vi "optimize swerve.vi"(8 "error in (no error)":errorcluster, 9 "current angle (deg)":dbl, 10 "target angle (deg)":dbl, 11 "velocity":dbl) -> (0 "error out":errorcluster, 1 "reset POS to ABS":bool, 2 "steer angle (deg)":dbl=-90.0, 3 "velocity":dbl)   [LabVIEW 2023]
uses:
  <vilib>/Analysis/coordinate.llb/Angle Units.ctl
  <vilib>/Analysis/coordinate.llb/Angle Range (Degree).ctl
  <vilib>/Analysis/coordinate.llb/Wrap Angle (scalar).vi
  <vilib>/Analysis/NI_AAL_Angle.lvlib
panel:
  out "invert V":bool
  out "angle to supp":dbl=-90.0
  out "angle to target":dbl=90.0
  out "supp angle":dbl=-90.0
  out "angle delta CCW":dbl=90.0
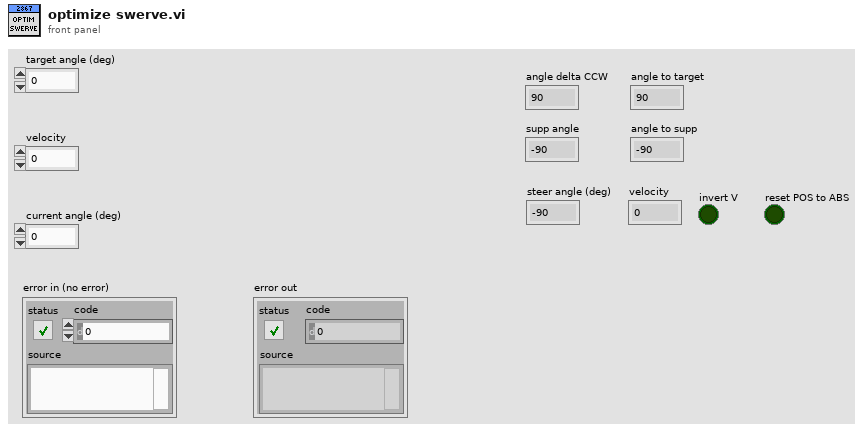
[diagram p1: front panel]
types:
  T1 = typedef "NI_AAL_Angle.lvlib/Angle Range (Degree).ctl" = u16
  T2 = typedef "NI_AAL_Angle.lvlib/Angle Units.ctl" = i32
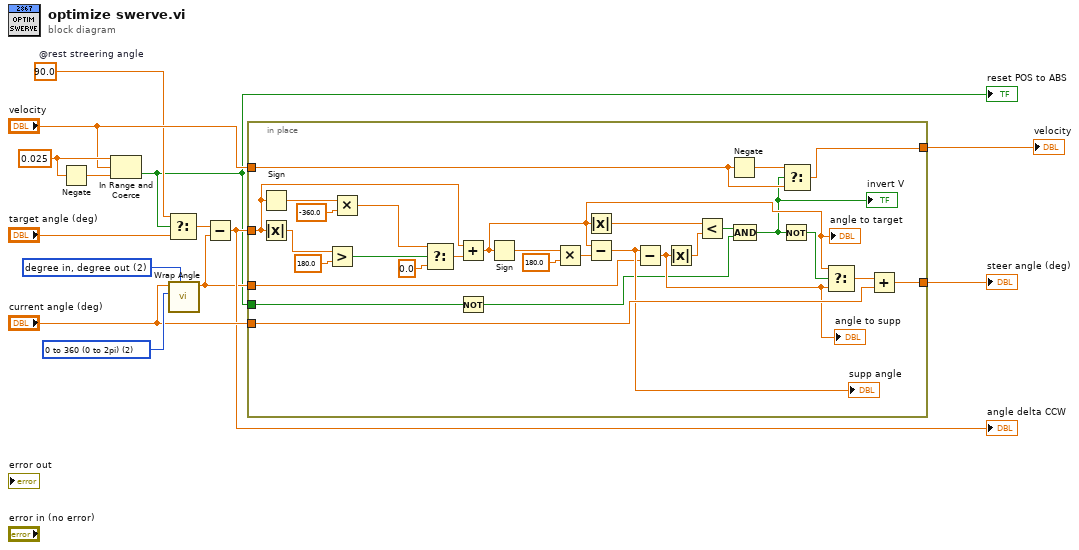
[diagram p0: block diagram]
diagram:
  w2 = 90.0  # @rest streering angle
  w5 = 0.025 ("upper limit")
  w12 = T1 2 items=["none", "-180 to 180 (-pi to pi)", "0 to 360 (0 to 2pi)"] ("angle range")
  w13 = T2 2 items=["radian in, radian out", "radian in, degree out", "degree in, degree out", "degree in, radian out"] ("angle units")
  n1 = Negate(x=w5) -> (-x=w4:dbl)
  n2 = In Range and Coerce(upper limit=w5, x="velocity", lower limit=w4) -> (In Range?=w1:bool)  [unwired: 1 out]
  "reset POS to ABS" <- w1
  n3 = Select(t=w2, s=w1, f="target angle (deg)") -> (s? t:f=w6:dbl)
  n4 = call-poly <vilib>:"Wrap Angle.vi"("angle units"=w13, "angle range"=w12, "angle in"="current angle (deg)") -> ("angle out"=w8:dbl)  [unwired: 7 in, 1 out]
  n5 = Subtract(x=w6, y=w8) -> (x-y=w10:dbl)
  "angle delta CCW" <- w10
  n6 = in-place {
    in-place-border: w10 -> [w38]
    in-place-border: "current angle (deg)" -> [w34]
    in-place-border: [w25] -> w14
    in-place-border: w8 -> [w31]
    in-place-border: [w21] -> w7
    in-place-border: "velocity" -> [w20]
    in-place-border: w1 -> [w18]
    n7 = Sign(1:w38) -> (0:w37:dbl)
    n8 = Absolute Value(x=w38) -> (abs(x)=w43:dbl)
    n9 = Greater?(x=w43, y=180.0) -> (0:w41:bool)
    n10 = Multiply(x=w37, y=-360.0 ("t")) -> (x*y=w36:dbl)
    n11 = Select(t=w36, s=w41, f=0.0) -> (s? t:f=w39:dbl)
    n12 = Add(x=w38, y=w39) -> (x+y=w24:dbl)
    "angle to target" <- w24
    n13 = Not(x=w18) -> (.not. x?=w17:bool)
    n14 = Sign(1:w24) -> (0:w29:dbl)
    n15 = Multiply(x=w29, y=180.0) -> (x*y=w30:dbl)
    n16 = Absolute Value(x=w24) -> (abs(x)=w23:dbl)
    n17 = Subtract(x=w24, y=w30) -> (x-y=w32:dbl)
    "supp angle" <- w32
    n18 = Subtract(x=w32, y=w31) -> (x-y=w27:dbl)
    "angle to supp" <- w27
    n19 = Absolute Value(x=w27) -> (abs(x)=w22:dbl)
    n20 = Less?(x=w23, y=w22) -> (x < y?=w28:bool)
    n21 = Negate(x=w20) -> (-x=w19:dbl)
    n22 = Compound Arithmetic op=AND(w28, w17) -> (w16:bool)
    "invert V" <- w16
    n23 = Not(x=w16) -> (.not. x?=w15:bool)
    n24 = Select(t=w19, s=w16, f=w20) -> (s? t:f=w21:dbl)
    n25 = Select(t=w24, s=w15, f=w27) -> (s? t:f=w26:dbl)
    n26 = Add(x=w26, y=w34) -> (x+y=w25:dbl)
  }
  "steer angle (deg)" <- w14
  "velocity" <- w7
